vi "dataset_connection_name.get.vi"(8 "error in (no error)":errorcluster, 11 "Nominal IO Client in":T1 format="%.0x") -> (0 "error out":errorcluster, 2 "dataset connection name":string, 3 "Nominal IO Client out":T1 format="%.0x", 4 "Found":bool)   [LabVIEW 2024, in "Nominal Client Scripting.lvlib"]
uses:
  Nominal Client Scripting.lvlib
  <vilib>/NI VeriStand/Custom Device API/Custom Device Item Ref.ctl
  <vilib>/NI VeriStand/Custom Device API/Get Item Property (String).vi
  <vilib>/NI VeriStand/Custom Device API/Custom Device API.lvlib
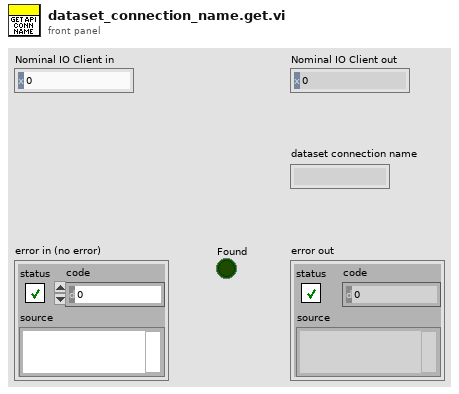
[diagram p1: front panel]
types:
  T1 = typedef "Custom Device API.lvlib/Custom Device Item Ref.ctl" = u64
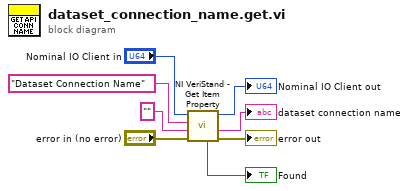
[diagram p0: block diagram]
diagram:
  n1 = call-poly <vilib>:"NI VeriStand - Get Item Property.vi"("error in (no error)"="error in (no error)", "Default Value"="", "Property Name"="Dataset Connection Name", "Item Ref in"="Nominal IO Client in") -> ("error out"=→"error out":errorcluster, "Value"=→"dataset connection name":string, "Item Ref out"=→"Nominal IO Client out":T1, "Found?"=→"Found":bool)  [unwired: 4 in]
